vi "wa32 ReadFile with Timeout.vi"(7 "timeout [ms]":i32=3000, 8 "error in (no error)":errorcluster, 10 "read count (0: all)":i32, 11 "pipe handle":i32) -> (0 "error out":errorcluster, 1 "read count":u32, 2 "data out":u8[](array[numeric]), 3 "pipe handle out":i32)   [LabVIEW 2020, in "GOLPI library.lvlib"]
doc: "Tries read pipe data using ReadFile with timeout. Use read count = 0 to read all data."
uses:
  GOLPI library.lvlib
  <vilib>/Utility/error.llb/Error Cluster From Error Code.vi
  <vilib>/ErrorRing/Error Ring.xnode
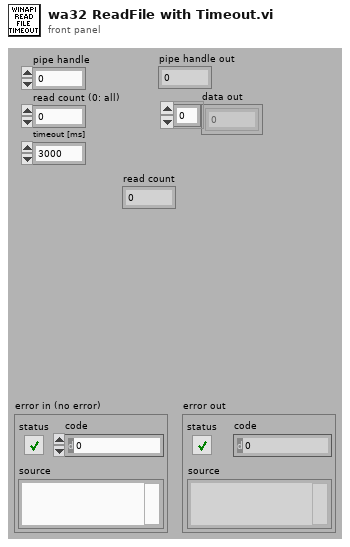
[diagram p1: front panel]
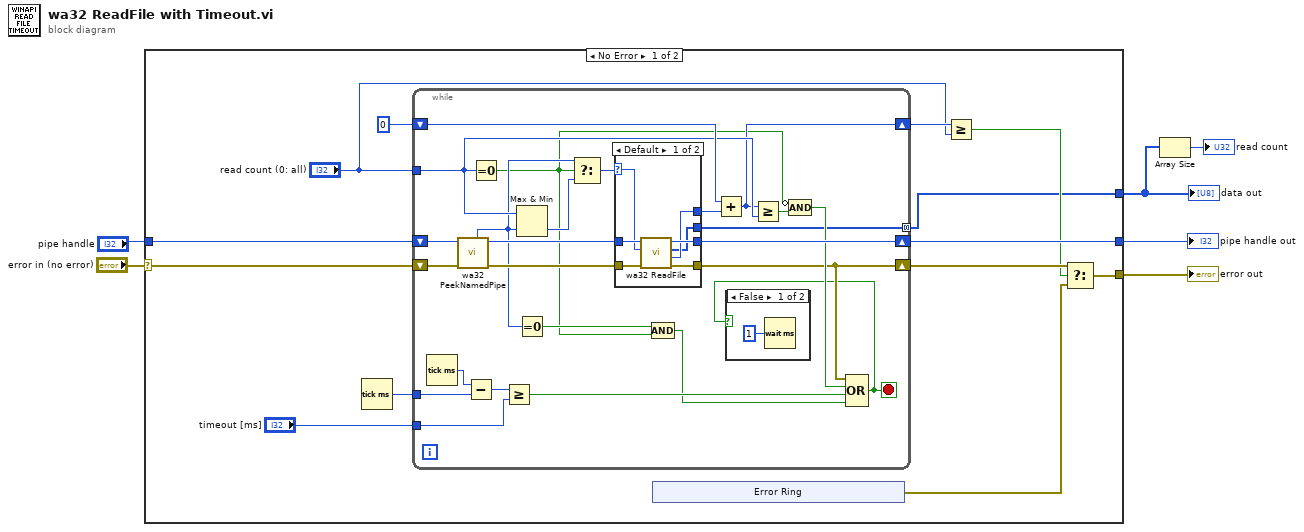
[diagram p0: block diagram]
diagram:
  n1 = case shown="No Error" "error in (no error)" {
    selector: "error in (no error)" -> [w16 w61]
    tunnel: [w18 w60] -> w6
    tunnel: [w17 w61] -> w5
    tunnel: "pipe handle" -> [w15 w60]
    tunnel: [w8 _] -> w1
    frame No Error {
      n2 = Tick Count (ms)() -> (millisecond timer value=w19:u32)
      n3 = while {
        shift-right: [w38] -> w18
        shift-left: w15 -> [w43]
        tunnel: "read count (0: all)" -> [w35]
        tunnel: w19 -> [w48]
        tunnel: "timeout [ms]" -> [w46]
        shift-right: [w30] -> w13
        shift-left: 0 -> [w37]
        shift-right: [w32] -> w11
        shift-left: w16 -> [w44]
        tunnel: [w31] -> w8 mode=concatenating
        stop <- w25 stop-if-true
        n4 = Tick Count (ms)() -> (millisecond timer value=w49:u32)
        n5 = call "wa32 PeekNamedPipe.vi"("error in"=w44, "handle"=w43) -> ("error out"=w41:errorcluster, "handle out"=w39:i32, "available bytes"=w28:u32)  [unwired: 4 in, 3 out]
        n6 = Subtract(x=w49, y=w48) -> (x-y=w47:u32)
        n7 = Equal To 0?(x=w35) -> (x = 0?=w27:bool)
        n8 = Greater Or Equal?(x=w47, y=w46) -> (x >= y?=w45:bool)
        n9 = Max & Min(x=w35, y=w28) -> (min(x,y)=w42:u32)  [unwired: 1 out]
        n10 = Equal To 0?(x=w28) -> (x = 0?=w29:bool)
        n11 = Select(t=w28, s=w27, f=w42) -> (s? t:f=w40:u32)
        n12 = case shown="Default" w40 {
          selector: w40 -> [w50 _]
          tunnel: w41 -> [w56 w57]
          tunnel: w39 -> [w55 w58]
          tunnel: [w54 w57] -> w32
          tunnel: [w53 w58] -> w38
          tunnel: [w52 _] -> w36
          tunnel: [w51 _] -> w31
          frame Default {
            n13 = call "wa32 ReadFile.vi"("error in"=w56, "bytes to read (0)"=w50, "handle"=w55) -> ("error out"=w54:errorcluster, "read bytes"=w52:u32, "read data"=w51:u8[], "handle out"=w53:i32)  [unwired: 4 in, 1 out]
          }
          frame 0 {
          }
        }
        n14 = Compound Arithmetic op=AND(w29, w27) -> (w26:bool)
        n15 = Add(x=w37, y=w36) -> (x+y=w30:u32)
        n16 = Greater Or Equal?(x=w30, y=w35) -> (x >= y?=w34:bool)
        n17 = Compound Arithmetic op=AND(invert w27, w34) -> (w33:bool)
        n18 = Compound Arithmetic op=OR(w32, w33, w45, w26) -> (w25:bool)
        n19 = case shown="False" w25 {
          frame False {
            n20 = Wait (ms)(milliseconds to wait=u32 1) -> ()  [unwired: 1 out]
          }
          frame True {
          }
        }
      }
      n21 = xnode "Error Ring"() -> ("error out"=w10:errorcluster)
      n22 = Greater Or Equal?(x=w13, y="read count (0: all)") -> (x >= y?=w9:bool)
      n23 = Select(t=w11, s=w9, f=w10) -> (s? t:f=w17:errorcluster)
    }
    frame Error {
    }
  }
  "error out" <- w5
  "pipe handle out" <- w6
  "data out" <- w1
  n24 = Array Size(array=w1) -> (size(s)=→"read count":i32)
